vi "Correct_Position_info_2021.vi"() -> (0 "error out":errorcluster, 4 "Path":path)   [LabVIEW 2020]
panel:
  in  "Instument Index":i32
  out "Array":path[](array[path])
  out "File Changed":bool
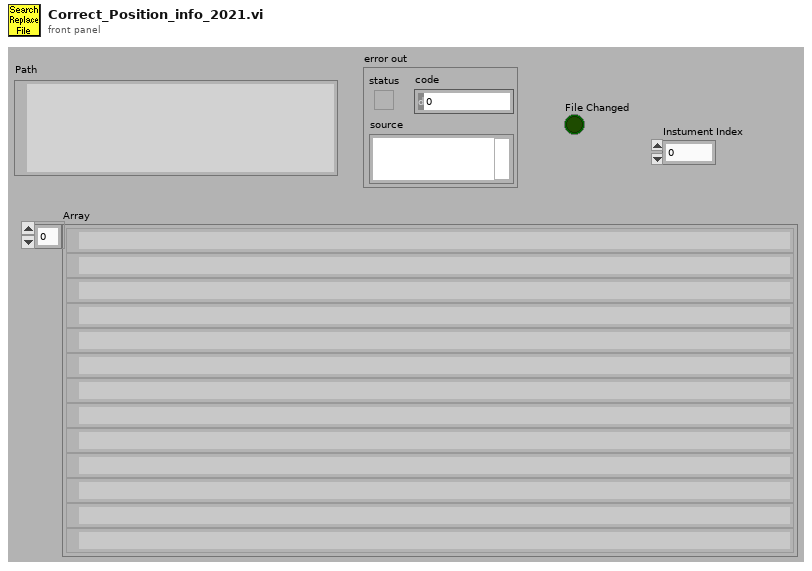
[diagram p1: front panel]
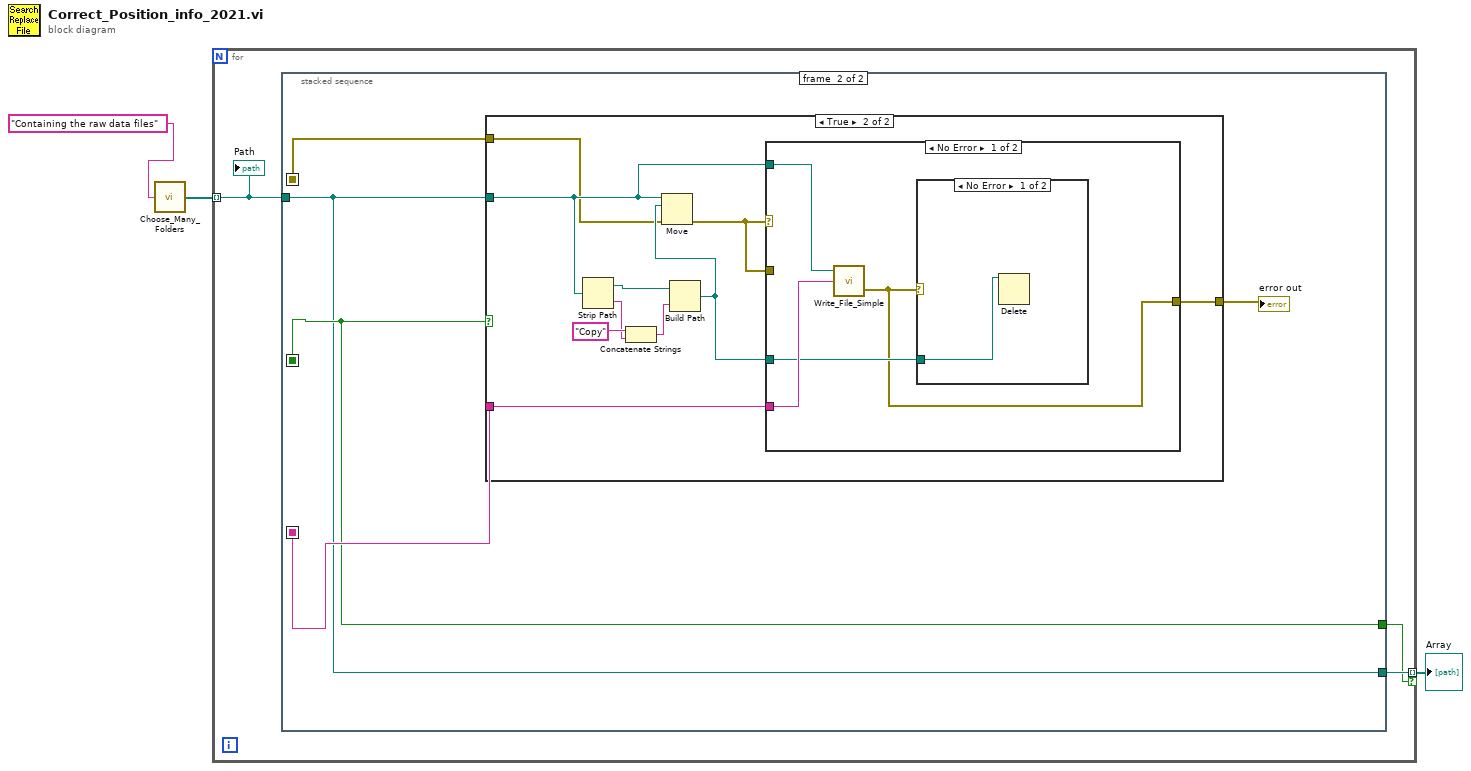
[diagram p0: block diagram]
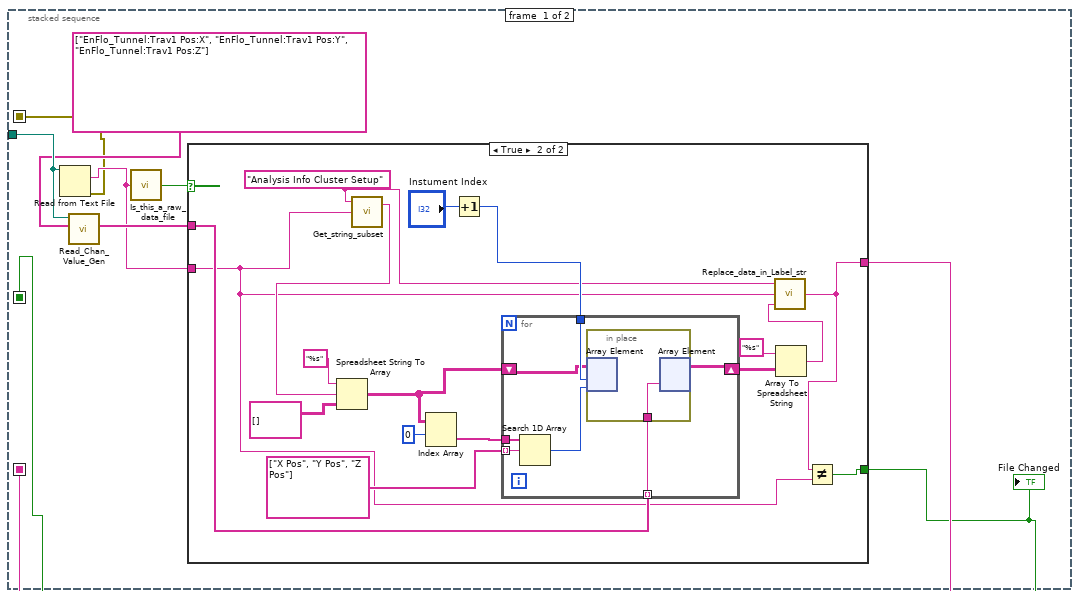
[diagram p2: hidden frame]
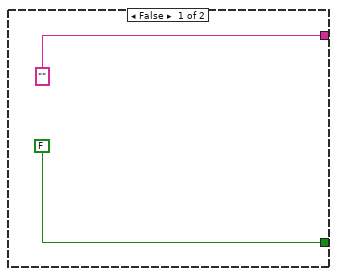
[diagram p3: hidden frame]
diagram:
  n1 = call "Choose_Many_Folders.vi"("Purpose of choosing folder"="Containing the raw data files") -> ("Files"=w2:path[])
  n2 = for {
    tunnel: w2 -> [w6] mode=indexing
    tunnel: [w5] -> w1 mode=indexing if=w4
    n3 = stacked-sequence {
      seq-local: [w7 _] -> [_ w45]
      seq-local: [w14 _] -> [_ w44]
      seq-local: [w13 _] -> [_ w43]
      tunnel: w6 -> [w12 w42]
      tunnel: [_ w42] -> w5
      tunnel: [_ w43] -> w4
      frame #0 {
        n4 = Read from Text File(file (use dialog)=w12) -> (text=w8:string, error out=w7:errorcluster)  [unwired: 3 in, 2 out]
        n5 = call "Read_Chan_Value_Gen.vi"("Desired Ch Names"=string[] ["EnFlo_Tunnel:Trav1 Pos:X", "EnFlo_Tunnel:Trav1 Pos:Y", "EnFlo_Tunnel:Trav1 Pos:Z"], "Raw data file"=w12) -> ("Values"=w11:string[])  [unwired: 9 in]
        n6 = call "Is_this_a_raw_data_file.vi"("character string"=w8) -> ("Raw Dat File?"=w9:bool)  [unwired: 2 out]
        n7 = case shown="True" w9 {
          tunnel: ["" ("string") w17] -> w14
          tunnel: [FALSE w19] -> w13
          tunnel: w11 -> [_ w24]
          tunnel: w8 -> [_ w18]
          frame False {
          }
          frame True {
            w23 = "Analysis Info Cluster Setup"
            n8 = call "Get_string_subset.vi"("String to split"=w18, "File Label"=w23) -> ("Output string"=w29:string)  [unwired: 2 in, 1 out]
            n9 = Spreadsheet String To Array(format string="%s", spreadsheet string=w29, array type (2D Dbl)=string[][] []) -> (array=w25:string[][])  [unwired: 1 in]
            n10 = Index Array(array=w25, index (row)=0) -> (element=w30:string[])  [unwired: 1 in]
            n11 = Increment(x="Instument Index") -> (x+1=w26:i32)
            n12 = for {
              tunnel: w30 -> [w40]
              tunnel: string[] ["X Pos", "Y Pos", "Z Pos"] -> [w39] mode=indexing
              tunnel: w26 -> [w37]
              shift-right: [w35] -> w22
              shift-left: w25 -> [w36]
              tunnel: w24 -> [w34] mode=indexing
              n13 = Search 1D Array(1D array=w40, element=w39) -> (index of element=w38:i32)  [unwired: 1 out]
              n14 = in-place {
                in-place-border: w34 -> [w41]
                n15 = in-place-array #1(w36, w37, w38) -> ()  [unwired: 1 out]
                n16 = in-place-array #1(w41) -> (w35:string[][])  [unwired: 2 out]
              }
            }
            n17 = Array To Spreadsheet String(array=w22, 3:"%s" ("format string")) -> (spreadsheet string=w20:string)  [unwired: 1 in]
            n18 = call "Replace_data_in_Label_str.vi"("New data string"=w20, "Input string"=w18, "Variable name"=w23) -> ("Appended string"=w17:string)
            n19 = Not Equal?(x=w17, y=w18) -> (x != y?=w19:bool)
          }
        }
        "File Changed" <- w13
      }
      frame #1 {
        n20 = case shown="True" w43 {
          tunnel: w42 -> [_ w53]
          tunnel: w44 -> [_ w52]
          tunnel: [w47 w50] -> w46
          tunnel: w45 -> [w47 w48]
          frame False {
          }
          frame True {
            n21 = Strip Path(path=w53) -> (stripped path=w54:path, name=w56:string)
            n22 = Concatenate Strings("Copy" ("name or relative path"), w56) -> (w55:string)
            n23 = Build Path(base path=w54, name or relative path=w55) -> (appended path=w51:path)
            n24 = Move(source path=w53, error in=w48, 10:w51) -> (error out=w49:errorcluster)  [unwired: 2 in, 2 out]
            n25 = case shown="No Error" w49 {
              tunnel: w53 -> [w61 _]
              tunnel: w52 -> [w60 _]
              tunnel: w51 -> [w59 _]
              tunnel: [w58 w63] -> w50
              tunnel: w49 -> [_ w63]
              frame No Error {
                n26 = call "Write_File_Simple.vi"("character string"=w60, "file path"=w61) -> ("error out"=w58:errorcluster)  [unwired: 1 in, 1 out]
                n27 = case shown="No Error" w58 {
                  tunnel: w59 -> [w62 _]
                  frame No Error {
                    n28 = Delete(path (use dialog)=w62) -> ()  [unwired: 4 in, 3 out]
                  }
                  frame Error {
                  }
                }
              }
              frame Error {
              }
            }
          }
        }
        "error out" <- w46
      }
    }
    "Path" <- w6
  }
  "Array" <- w1
